vi "Load_Destinations.vi"(8 "error in (no error)":errorcluster, 11 "AB_PackedLibrary in":refnum<class "AB_PackedLibrary.lvclass">) -> (0 "error out":errorcluster, 3 "AB_PackedLibrary out":refnum<class "AB_PackedLibrary.lvclass">)   [LabVIEW 2020, in "AB_PackedLibrary.lvclass"]
uses:
  <vilib>/AppBuilder/AB_Classes/PackedLib/AB_PackedLibrary.lvclass
  e:/builds/penguin/labview/branches/2020/dev/dist/vi.lib/AppBuilder/AB_Classes/Build/AB_Build.lvclass
  <vilib>/AppBuilder/AB_Classes/TargetFile/AB_Targetfile.lvclass
  <vilib>/AppBuilder/AB_Classes/Build/AB_Build.lvclass
  <vilib>/AppBuilder/AB_Classes/Destination/AB_Destination.lvclass
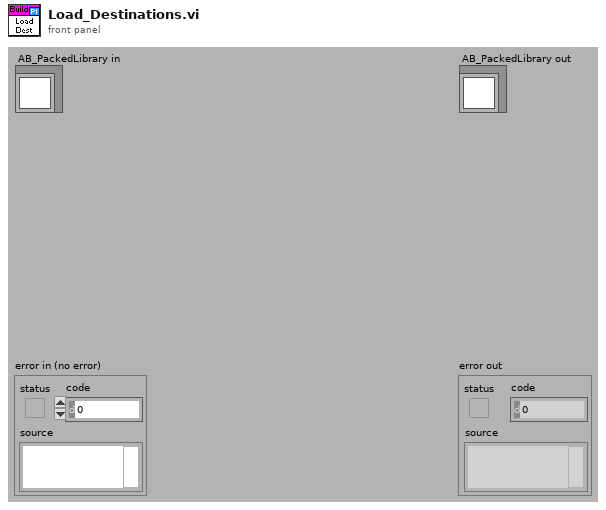
[diagram p1: front panel]
types:
  T1 = typedef "AB_Build.ctl" = cluster{"buildSpecName":string, "buildSpecDescription":string, "destinations":refnum<class "AB_Destination.lvclass">[], "exclusionOption":T2, "defaultLanguage":string, "supportedLanguages":string[], "excludedDirectories":path[], "buildContext":refnum<vi>, "buildObject":T3, "preview":bool, "programatic":bool, "progressBarEvents":T4, "userLog_Path":path, "preActionID":string, "preAction_Path":path, "postActionID":string, "postAction_Path":path, "eng_checkForBrokenVIs?":bool, "eng_verboseLinkerErrors?":bool, "localDest_Path":path, "targetDest_Path":path, "removeVIObject":u16, "cache":refnum<class "PreviewCache.lvclass">, "use cache":bool, "previewCache_ID":string, "buildCache_ID":string, "eng_TempLocalDest_Path":path, "eng_collectDependencies?":bool, "versionInfo":cluster{"buildVersion":cluster{"major":u16, "minor":u16, "patch":u16, "build":u16}, "autoIncrement":bool}, "eng_enableVIChecksums":bool}
  T2 = typedef "AB_Exclusion_Option.ctl" = cluster{"typedefs":bool, "polymorphicVIs":bool, "unusedLibraryItems":bool, "modifyLibraryFile":bool, "edit-timeDependencies":bool, "inlineVIs":bool, "dependent PPLs":bool, "dependent DLLs":bool}
  T3 = typedef "ItemRef.ctl" = u64
  T4 = typedef "provcom_ProgressBar_Events.ctl" = cluster{"newJob":refnum<user-event>, "newItem":refnum<user-event>, "errorMsg":T5, "cancel":refnum<user-event>}
  T5 = typedef "mxLvBuildError.ctl" = refnum<user-event>
  T6 = typedef "AB_Destination.ctl" = cluster{"destName":string, "path":path, "libraryName":string, "preserveHierarchy":bool, "eng_inBuild":bool, "eng_libraryReference":refnum<vi>, "eng_restictAddToNewLibrary":bool}
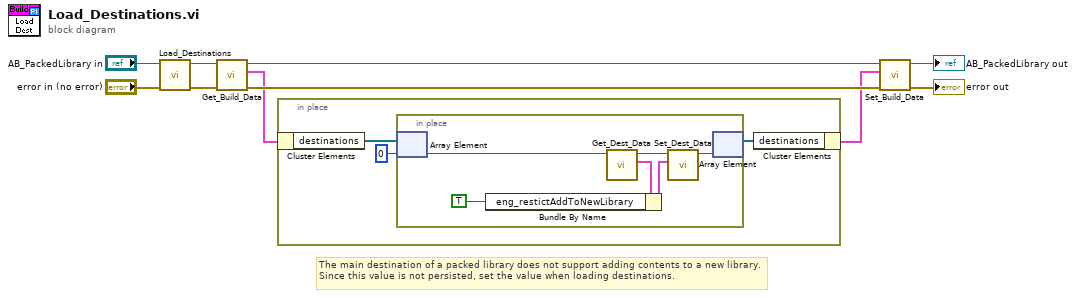
[diagram p0: block diagram]
diagram:
  # "The main destination of a packed library does not support adding contents to a new library. Since this value is not persisted, set the value when loading destinations."
  n1 = call-parent "Load_Destinations.vi"("error in (no error)"="error in (no error)", "AB_Build in"="AB_PackedLibrary in") -> ("error out"=w7:errorcluster, "AB_Build out"=w8:refnum<class "AB_PackedLibrary.lvclass">)  [unwired: 8 in]
  n2 = call <vilib>:"Get_Build_Data.vi"("error in (no error)"=w7, "Class in"=w8) -> ("error out"=w4:errorcluster, "data"=w2:T1, "Class out"=w6:refnum<class "AB_PackedLibrary.lvclass">)  [unwired: 7 in]
  n3 = in-place {
    n4 = in-place-cluster #1(w2) -> ("destinations"=w11:refnum<class "AB_Destination.lvclass">[])
    n5 = in-place {
      n6 = in-place-array #2(w11, 0) -> (w18:refnum<class "AB_Destination.lvclass">)
      n7 = call <vilib>:"Get_Dest_Data.vi"("Class in"=w18) -> ("destName"=w16:T6, "Class out"=w19:refnum<class "AB_Destination.lvclass">)  [unwired: 8 in, 1 out]
      n8 = Bundle By Name(cluster=w16, "eng_restictAddToNewLibrary"=TRUE) -> (w15:T6)
      n9 = call <vilib>:"Set_Dest_Data.vi"("destName"=w15, "Class in"=w19) -> ("Class out"=w17:refnum<class "AB_Destination.lvclass">)  [unwired: 8 in, 1 out]
      n10 = in-place-array #2(w17) -> (w12:refnum<class "AB_Destination.lvclass">[])  [unwired: 1 out]
    }
    n11 = in-place-cluster #1("destinations"=w12) -> (w1:T1)
  }
  n12 = call <vilib>:"Set_Build_Data.vi"("error in (no error)"=w4, "data"=w1, "Class in"=w6) -> ("error out"=→"error out":errorcluster, "Class out"=→"AB_PackedLibrary out":refnum<class "AB_PackedLibrary.lvclass">)  [unwired: 7 in]
